vi "Pre-Build Action.vi"(6 "Top Level/Always Included VIs":path[](array[path]), 7 "Main Destination Path":path, 9 "Target Name":string, 10 "Build Specification Name":string, 11 "Project Path":path) -> (0 "error out":errorcluster)   [LabVIEW 2024]
uses:
  <vilib>/Utility/error.llb/Error Cluster From Error Code.vi
  <vilib>/ErrorRing/Error Ring.xnode
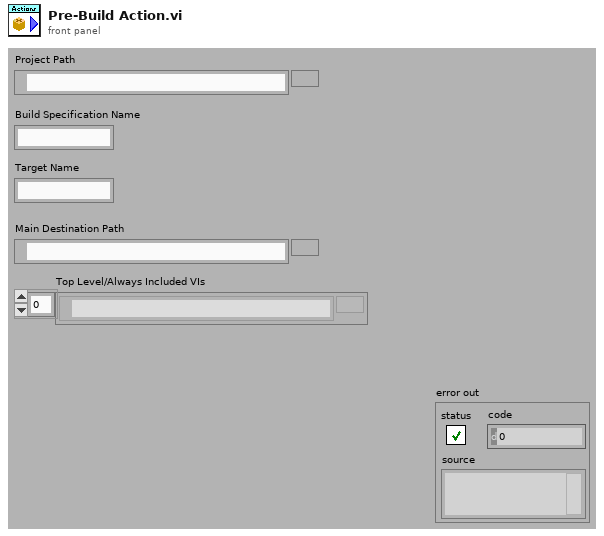
[diagram p1: front panel]
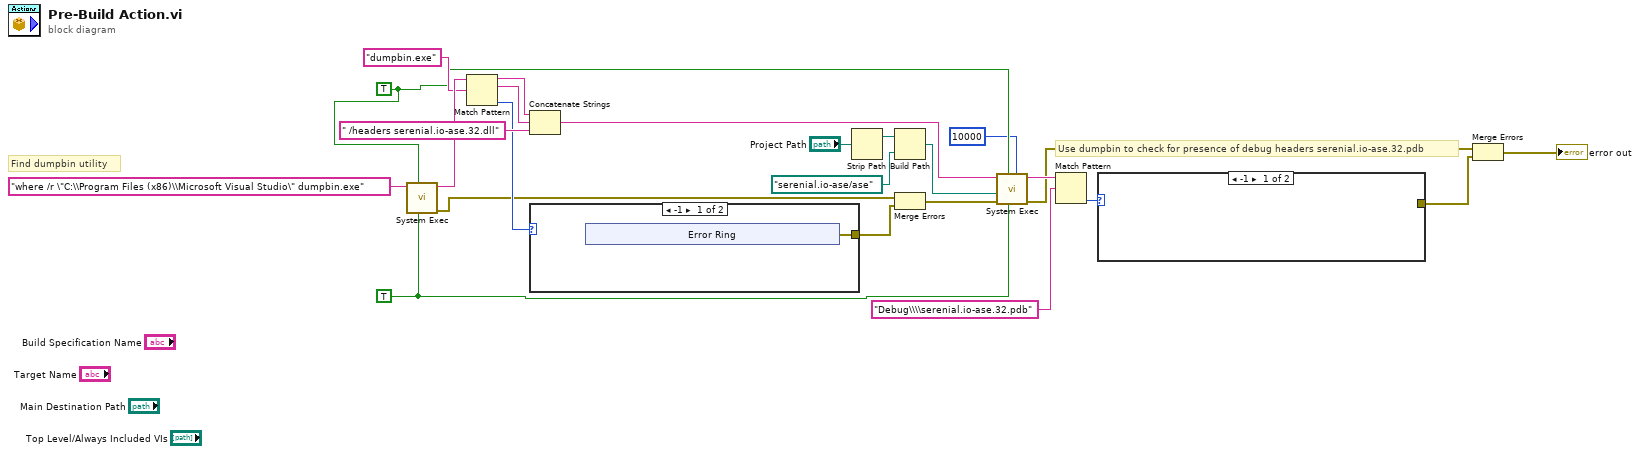
[diagram p0: block diagram]
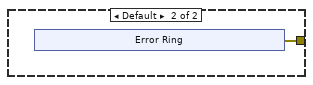
[diagram p3: hidden frame]
diagram:
  w16 = TRUE ("run minimized? (F)")
  w17 = TRUE ("wait until completion? (T)")
  # "Find dumpbin utility"
  # "Use dumpbin to check for presence of debug headers serenial.io-ase.32.pdb"
  n1 = call <vilib>:"System Exec.vi"("run minimized? (F)"=w16, "wait until completion? (T)"=w17, "command line"="where /r \"C:\\Program Files (x86)\\Microsoft Visual Studio\" dumpbin.exe") -> ("error out"=w5:errorcluster, "standard output"=w23:string)  [unwired: 5 in, 2 out]
  n2 = Match Pattern(string=w23, regular expression="dumpbin.exe") -> (before substring=w7:string, match substring=w8:string, offset past match=w6:i32)  [unwired: 1 in, 1 out]
  n3 = Concatenate Strings(w7, w8, " /headers serenial.io-ase.32.dll" ("format string")) -> (w18:string)
  n4 = case shown="-1" w6 {
    tunnel: [w25 _] -> w4
    frame -1 {
      n5 = xnode "Error Ring"() -> ("error out"=w25:errorcluster)
    }
    frame Default {
    }
  }
  n6 = Strip Path(path="Project Path") -> (stripped path=w20:path)  [unwired: 1 out]
  n7 = Build Path(base path=w20, name or relative path=path "serenial.io-ase/ase") -> (appended path=w2:path)
  n8 = Merge Errors(w5, w4) -> (w3:errorcluster)
  n9 = call <vilib>:"System Exec.vi"("expected output size  (4096)"=u32 10000, "run minimized? (F)"=w16, "wait until completion? (T)"=w17, "error in (no error)"=w3, "working directory"=w2, "command line"=w18) -> ("error out"=w10:errorcluster, "standard output"=w13:string)  [unwired: 2 in, 2 out]
  n10 = Match Pattern(string=w13, regular expression="Debug\\\\serenial.io-ase.32.pdb") -> (offset past match=w11:i32)  [unwired: 1 in, 3 out]
  n11 = case shown="-1" w11 {
    tunnel: [_ w31] -> w9
    frame -1 {
    }
    frame Default {
      n12 = xnode "Error Ring"() -> ("error out"=w31:errorcluster)
    }
  }
  n13 = Merge Errors(w10, w9) -> (→"error out":errorcluster)
